vi "Evaluate Analog Edge Trigger (Array).vi"(8 "error in (no error)":errorcluster, 10 "Trigger Data":dbl[](array[numeric]), 11 "Analog Edge Trigger in":refnum<class "Analog Edge Trigger.lvclass">) -> (0 "error out":errorcluster, 1 "Trigger indices":i32[](array[numeric]), 2 "Trigger":bool, 3 "Analog Edge Trigger out":refnum<class "Analog Edge Trigger.lvclass">)   [LabVIEW 2015, in "Waveform Data Logger Engine.lvlib" / "Analog Edge Trigger.lvclass"]
uses:
  Analog Edge Trigger.lvclass
  Analog Edge Trigger.lvclass/Analog Edge Trigger.ctl
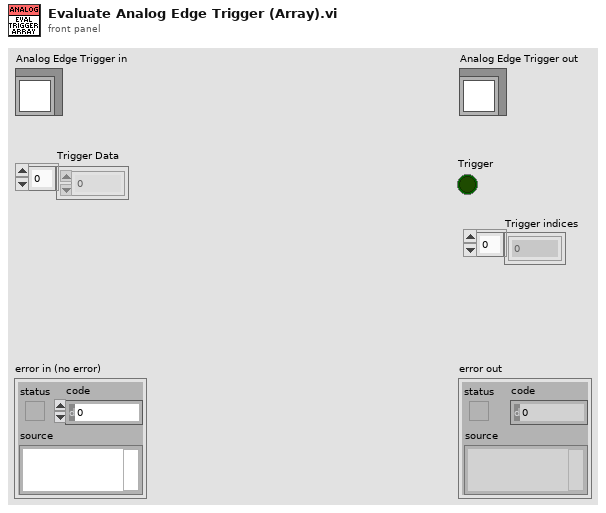
[diagram p1: front panel]
types:
  T1 = typedef "Waveform Data Logger Engine.lvlib/Analog Edge Trigger.lvclass/Analog Slope Type.ctl" = enum16{"Rising", "Falling"}
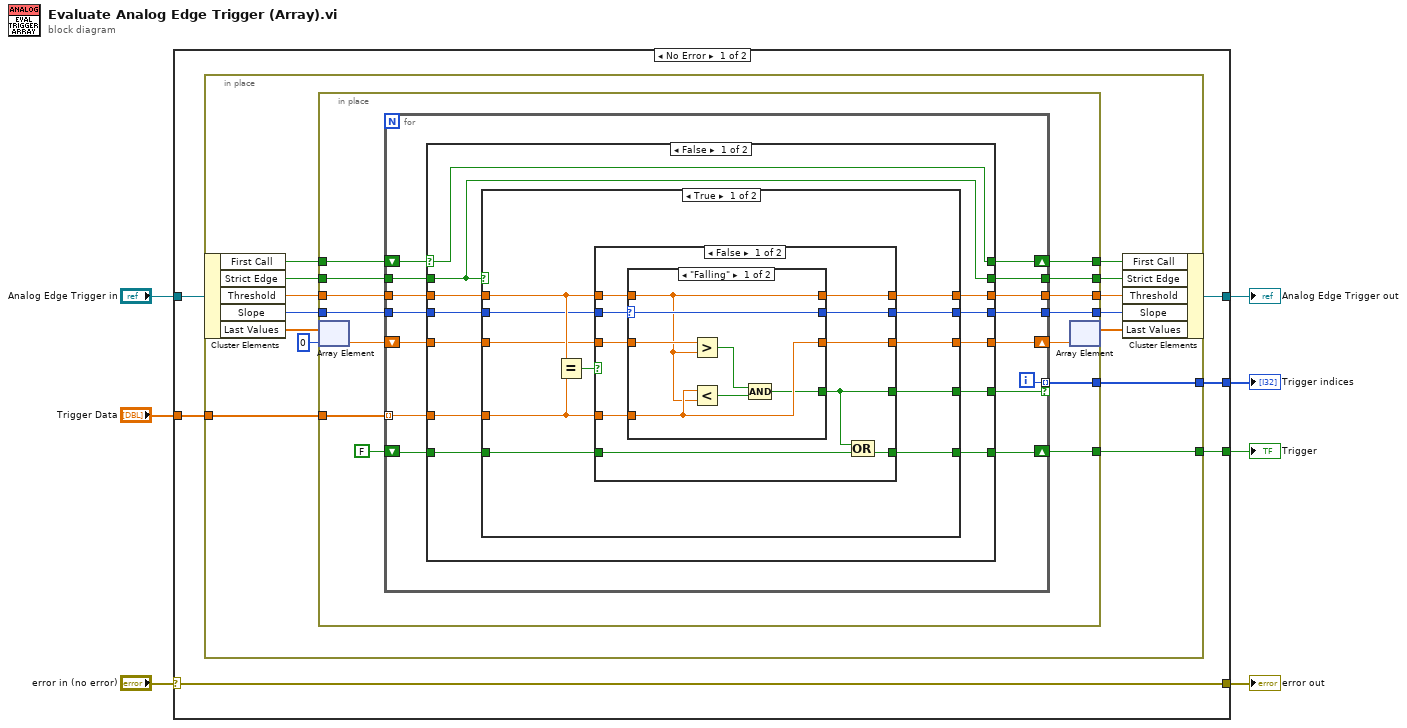
[diagram p0: block diagram]
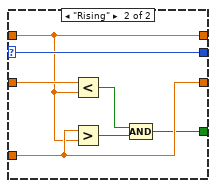
[diagram p2: hidden frame]
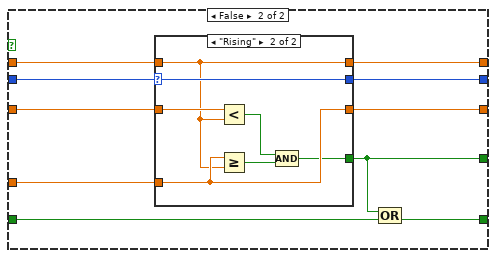
[diagram p4: hidden frame]
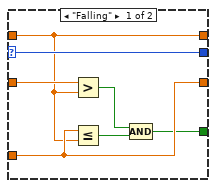
[diagram p5: hidden frame]
diagram:
  n1 = case shown="No Error" "error in (no error)" {
    selector: "error in (no error)" -> [w9 w138]
    tunnel: "Analog Edge Trigger in" -> [w13 w137]
    tunnel: "Trigger Data" -> [w12 _]
    tunnel: [w11 _] -> w5
    tunnel: [w10 w137] -> w4
    tunnel: [w9 w138] -> w2
    tunnel: [w8 _] -> w1
    frame No Error {
      n2 = in-place {
        in-place-border: w12 -> [w21]
        in-place-border: [w18] -> w11
        in-place-border: [w17] -> w8
        n3 = in-place-cluster #1(w13) -> ("First Call"=w23:bool, "Strict Edge"=w20:bool, "Threshold"=w26:dbl, "Slope"=w24:T1, "Last Values"=w16:dbl[])
        n4 = in-place {
          in-place-border: [w41] -> w27
          in-place-border: w26 -> [w40]
          in-place-border: [w39] -> w25
          in-place-border: w24 -> [w38]
          in-place-border: w23 -> [w37]
          in-place-border: [w36] -> w22
          in-place-border: w21 -> [w35]
          in-place-border: w20 -> [w34]
          in-place-border: [w33] -> w19
          in-place-border: [w31] -> w18
          in-place-border: [w30] -> w17
          n5 = in-place-array #2(w16, 0) -> (w29:dbl)
          n6 = for {
            tunnel: [w56] -> w41
            tunnel: w40 -> [w55]
            tunnel: [w54] -> w39
            tunnel: w38 -> [w53]
            tunnel: w35 -> [w48] mode=indexing
            tunnel: w34 -> [w47]
            tunnel: [w46] -> w33
            shift-right: [w51] -> w28
            shift-left: w29 -> [w52]
            shift-right: [w43] -> w31
            shift-left: FALSE -> [w45]
            tunnel: [w44] -> w30 mode=indexing if=w42
            shift-right: [w49] -> w36
            shift-left: w37 -> [w50]
            i -> [w44]
            n7 = case shown="False" w50 {
              selector: w50 -> [w60 _]
              tunnel: [w68 w136] -> w56
              tunnel: w55 -> [w67 w136]
              tunnel: [w66 w135] -> w54
              tunnel: w53 -> [w65 w135]
              tunnel: w52 -> [w64 _]
              tunnel: [w63 w134] -> w51
              tunnel: [w62 w132] -> w43
              tunnel: w48 -> [w61 w134]
              tunnel: [w60 _] -> w49
              tunnel: w47 -> [w59 w133]
              tunnel: [w59 w133] -> w46
              tunnel: w45 -> [w58 w132]
              tunnel: [w57 _] -> w42
              frame False {
                n8 = case shown="True" w59 {
                  tunnel: [w79 w117] -> w68
                  tunnel: w67 -> [w78 w116]
                  tunnel: [w77 w115] -> w66
                  tunnel: w65 -> [w76 w114]
                  tunnel: w64 -> [w75 w113]
                  tunnel: [w74 w112] -> w63
                  tunnel: [w73 w111] -> w62
                  tunnel: w61 -> [w72 w110]
                  tunnel: w58 -> [w70 w109]
                  tunnel: [w69 w108] -> w57
                  frame True {
                    n9 = Equal?(x=w78, y=w72) -> (x = y?=w71:bool)
                    n10 = case shown="False" w71 {
                      tunnel: [w83 w107] -> w79
                      tunnel: w78 -> [w88 w107]
                      tunnel: [w84 w106] -> w77
                      tunnel: w76 -> [w89 w106]
                      tunnel: w75 -> [w87 w105]
                      tunnel: [w85 w105] -> w74
                      tunnel: [w82 w104] -> w73
                      tunnel: w72 -> [w86 _]
                      tunnel: w70 -> [w81 w104]
                      tunnel: [w80 _] -> w69
                      frame False {
                        n11 = case shown="\"Falling\"" w89 {
                          selector: w89 -> [w92 w99]
                          tunnel: w88 -> [w91 w98]
                          tunnel: w87 -> [w96 w103]
                          tunnel: w86 -> [w93 w100]
                          tunnel: [w93 w100] -> w85
                          tunnel: [w92 w99] -> w84
                          tunnel: [w91 w98] -> w83
                          tunnel: [w90 w97] -> w80
                          frame "Falling" {
                            n12 = Greater?(x=w96, y=w91) -> (0:w95:bool)
                            n13 = Less?(x=w93, y=w91) -> (x < y?=w94:bool)
                            n14 = Compound Arithmetic op=AND(w95, w94) -> (w90:bool)
                          }
                          frame "Rising" {
                            n15 = Less?(x=w103, y=w98) -> (x < y?=w102:bool)
                            n16 = Greater?(x=w100, y=w98) -> (0:w101:bool)
                            n17 = Compound Arithmetic op=AND(w102, w101) -> (w97:bool)
                          }
                        }
                        n18 = Compound Arithmetic op=OR(w80, w81) -> (w82:bool)
                      }
                      frame True {
                        # "Do not keep track of values that are exactly equal to the threshold, so that we can tell if a previous value was actually above or below that threshold."
                      }
                    }
                  }
                  frame False {
                    n19 = case shown="\"Rising\"" w114 {
                      selector: w114 -> [w120 w127]
                      tunnel: w116 -> [w119 w126]
                      tunnel: w113 -> [w124 w131]
                      tunnel: w110 -> [w121 w128]
                      tunnel: [w121 w128] -> w112
                      tunnel: [w120 w127] -> w115
                      tunnel: [w119 w126] -> w117
                      tunnel: [w118 w125] -> w108
                      frame "Falling" {
                        n20 = Greater?(x=w124, y=w119) -> (0:w123:bool)
                        n21 = Less Or Equal?(x=w121, y=w119) -> (x <= y?=w122:bool)
                        n22 = Compound Arithmetic op=AND(w123, w122) -> (w118:bool)
                      }
                      frame "Rising" {
                        n23 = Less?(x=w131, y=w126) -> (x < y?=w130:bool)
                        n24 = Greater Or Equal?(x=w128, y=w126) -> (x >= y?=w129:bool)
                        n25 = Compound Arithmetic op=AND(w130, w129) -> (w125:bool)
                      }
                    }
                    n26 = Compound Arithmetic op=OR(w108, w109) -> (w111:bool)
                  }
                }
              }
              frame True {
                # "Just latch the trigger value on the first call. The trigger takes at least two timesteps to trigger."
              }
            }
          }
          n27 = in-place-array #2(w28) -> (w15:dbl[])  [unwired: 1 out]
        }
        n28 = in-place-cluster #1("First Call"=w22, "Strict Edge"=w19, "Threshold"=w27, "Slope"=w25, "Last Values"=w15) -> (w10:refnum<class "Analog Edge Trigger.lvclass">)
      }
    }
    frame Error {
    }
  }
  "error out" <- w2
  "Analog Edge Trigger out" <- w4
  "Trigger" <- w5
  "Trigger indices" <- w1
